vi "mergeDotNetPropNode.vi"   [LabVIEW 2020]
doc: "Gets (reads) and/or sets (writes) properties of a reference."
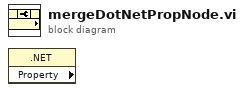
[diagram p0: block diagram]
diagram:
  n1 = property class=".NET" props=[]() -> ()  [unwired: 2 in, 3 out]
